vi "TeachAndPlay.vi"() -> ()   [LabVIEW 2013]
uses:
  ROS/Code/JointPositions.ctl
  ROS/Code/SubVIs/BaxterSide.ctl
  ROS/Code/SubVIs/BaxterButtons.ctl
  BaxterVIs/Command_Joint_Angles_cluster.vi
panel:
  in  "Idle Ctr 2":i32=1070
  in  "ITB Cluster":cluster{i16, i16, i16, i16}
  in  "Idle Ctr":i32=411
  in  "Right Path":T2(array[cluster])=[{"Position"={"e0"=0.0, "e1"=90.0, "s0"=50.0, "s1"=0.0, "w0"=0.0, "w1"=0.0, "w2"=0.0}, "Name"="Position0", "Gripper"=FALSE}, {"Position"={"e0"=0.0, "e1"=90.0, "s0"=30.0, "s1"=0.0, "w0"=0.0, "w1"=0.0, "w2"=0.0}, "Name"="Drop", "Gripper"=FALSE}] {"Position"."w2" scale=-175.25..175.25; "Position"."w1" scale=-90.0..120.0; "Position"."w0" scale=-175.25..175.25; "Position"."e1" scale=-3.0..150.0; "Position"."e0" scale=-173.5..173.5; "Position"."s1" scale=-123.0..60.0; "Position"."s0" scale=-141.0..51.0}
  in  "Functions":i32[](listbox)=[0, 1, 4, 5]
  out "Gripper State":bool
  in  "Left Path":T2(array[cluster])=[{"Position"={"e0"=0.0, "e1"=90.0, "s0"=-30.0, "s1"=0.0, "w0"=0.0, "w1"=0.0, "w2"=0.0}, "Name"="Position0", "Gripper"=FALSE}, {"Position"={"e0"=0.0, "e1"=90.0, "s0"=-50.0, "s1"=0.0, "w0"=0.0, "w1"=0.0, "w2"=0.0}, "Name"="Drop", "Gripper"=FALSE}] {"Position"."w2" scale=-175.25..175.25; "Position"."w1" scale=-90.0..120.0; "Position"."w0" scale=-175.25..175.25; "Position"."e1" scale=-3.0..150.0; "Position"."e0" scale=-173.5..173.5; "Position"."s1" scale=-123.0..60.0; "Position"."s0" scale=-141.0..51.0}
  in  "Tab":T3(tab)=enum."Play"
  in  "New Path?":bool
  out "Last Activity":string="Initializing"
  in  "Side":T4=enum."right"
  in  "New Path?":bool
  out "Last Activity":string="Initializing"
  in  "Settle":bool
  in  "Resend Right":bool
  in  "Resend Left":bool
  in  "Tolerance":dbl=1.0
  in  "Settle Time":u32=1000
  in  "Loop?":bool
  in  "Execution":T5(radio)
  in  "Left Step":i32
  in  "Right Step":i32
  in  "Same?":bool
  in  "right save path":path=path "C:/Program Files/Labview/user.lib/ROSforLV_0.1/Devices/Baxter/Baxter Examples/Paths/Tsai2RightW2.csv"
  in  "left save path":path=path "C:/Program Files/Labview/user.lib/ROSforLV_0.1/Devices/Baxter/Baxter Examples/Paths/TsaiLeftW2.csv"
  in  "Save":bool
  in  "left load file":path=path "C:/Program Files/Labview/user.lib/ROSforLV_0.1/Devices/Baxter/Baxter Examples/Paths/TsaiLeftS0.csv"
  in  "Load":bool
  in  "right load file":path=path "C:/Program Files/Labview/user.lib/ROSforLV_0.1/Devices/Baxter/Baxter Examples/Paths/Tsai2RightS0.csv"
  in  "stop":bool
  # "Not yet"
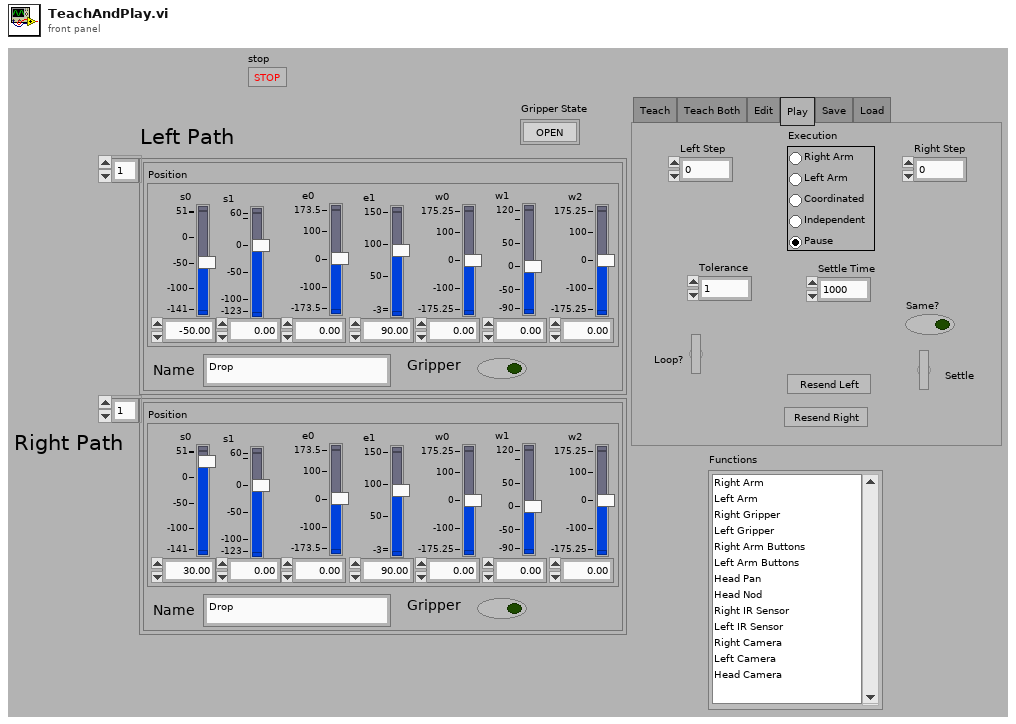
[diagram p1: front panel]
types:
  T1 = typedef "JointPositions.ctl" = cluster{"e0":dbl, "e1":dbl, "s0":dbl, "s1":dbl, "w0":dbl, "w1":dbl, "w2":dbl}
  T2 = cluster{"Position":T1, "Name":string, "Gripper":bool}[]
  T3 = enum32{"Teach", "Teach Both", "Edit", "Play", "Save", "Load"}
  T4 = typedef "BaxterSide.ctl" = enum16{"left", "right"}
  T5 = enum32{"Pause", "Right Arm", "Left Arm", "Coordinated", "Independent"}
  T6 = cluster{"Positions":T1, "Name":string, "Gripper":bool}
  T7 = enum16{"open", "replace", "create", "open or create", "replace or create", "replace or create with confirmation"}
  T8 = typedef "BaxterButtons.ctl" = u16
  T9 = cluster{"Cancel":bool, "OK":bool, "Show":bool, "Wheel":u8}
  T10 = cluster{"Positions":T1, "Name":string, "Gripper":bool}[]
  T11 = cluster{"Position":T1, "Name":string, "Gripper":bool}
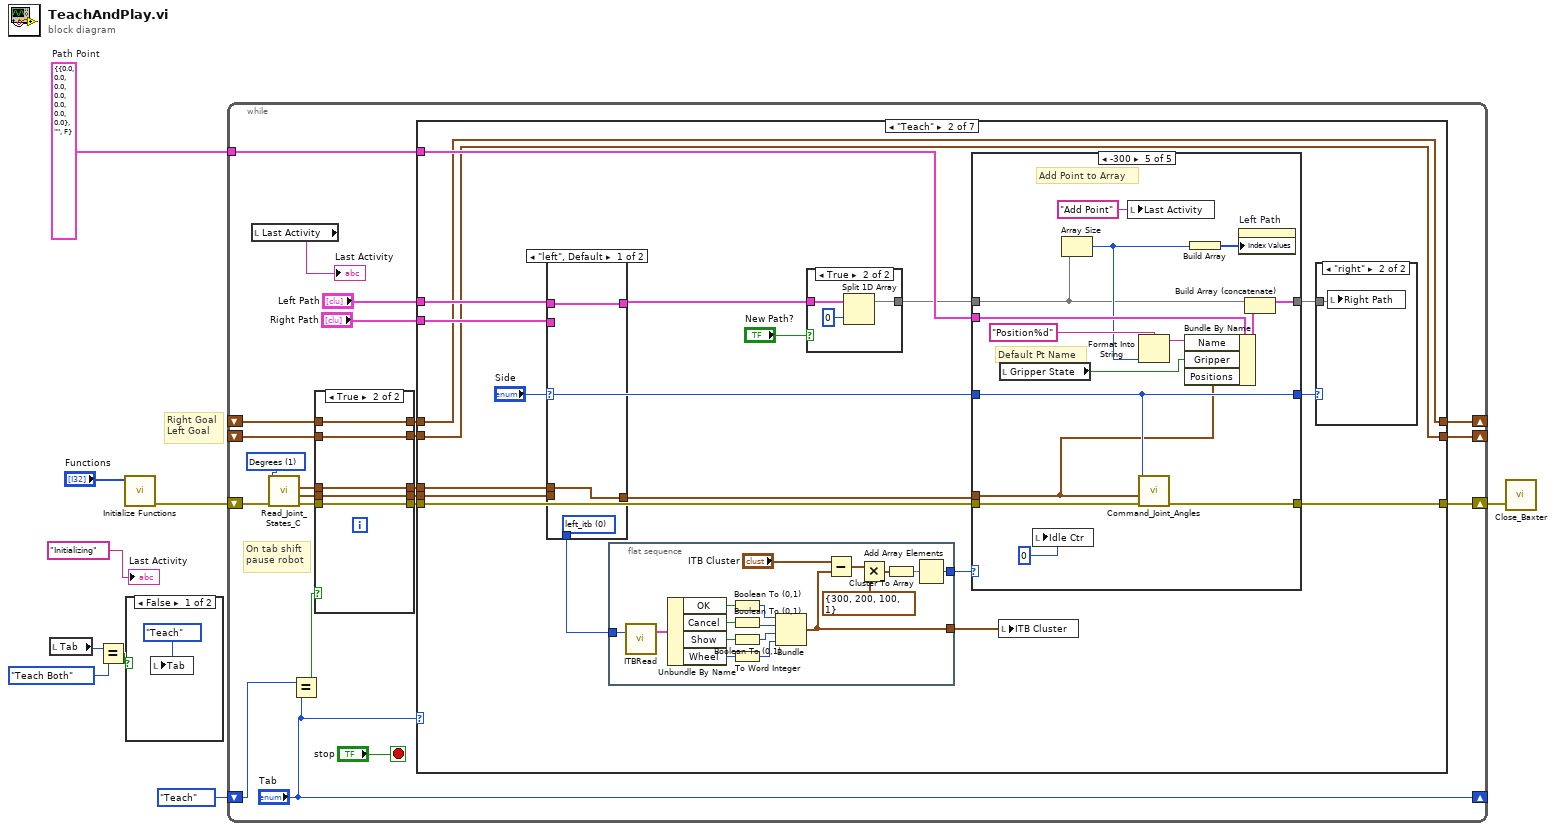
[diagram p0: block diagram]
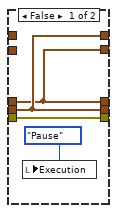
[diagram p3: hidden frame]
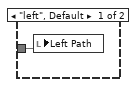
[diagram p5: hidden frame]
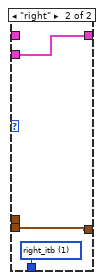
[diagram p6: hidden frame]
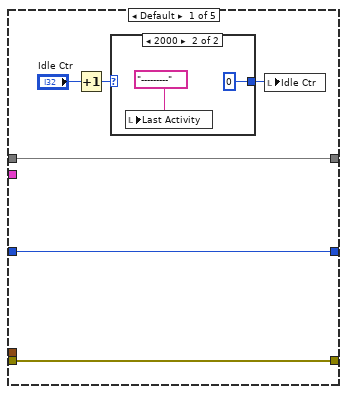
[diagram p8: hidden frame]
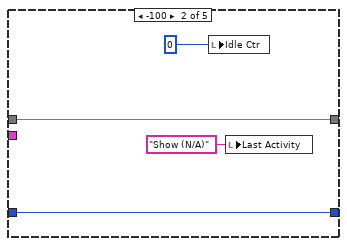
[diagram p10: hidden frame]
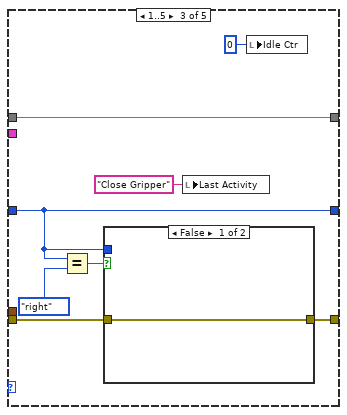
[diagram p11: hidden frame]
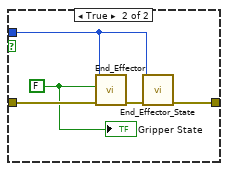
[diagram p12: hidden frame]
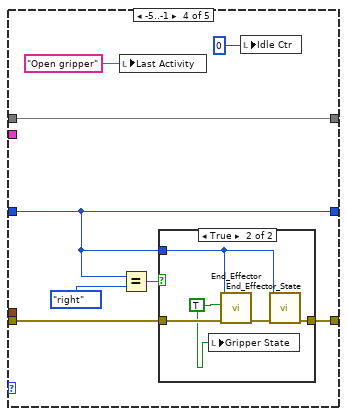
[diagram p13: hidden frame]
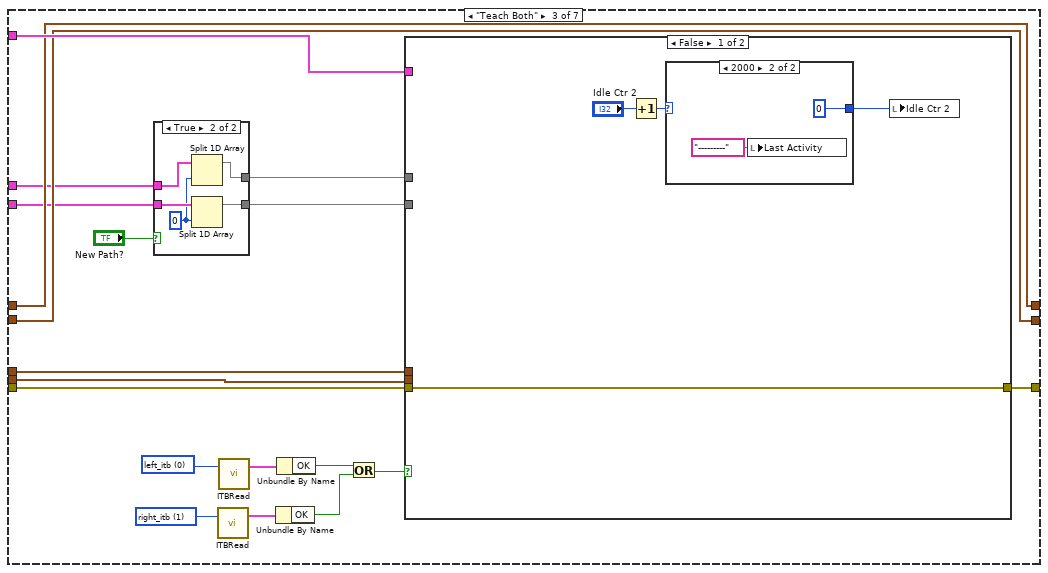
[diagram p15: hidden frame]
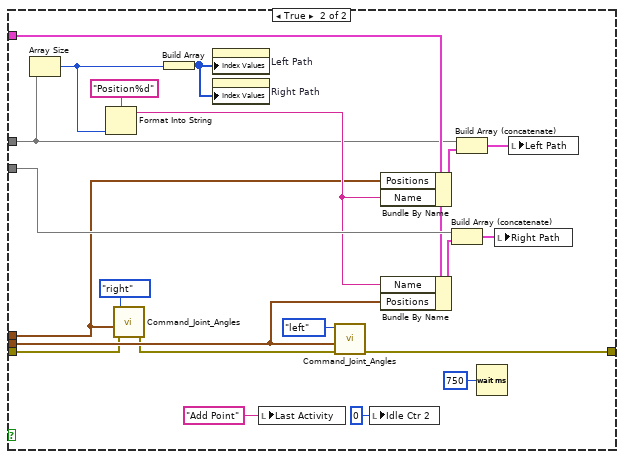
[diagram p18: hidden frame]
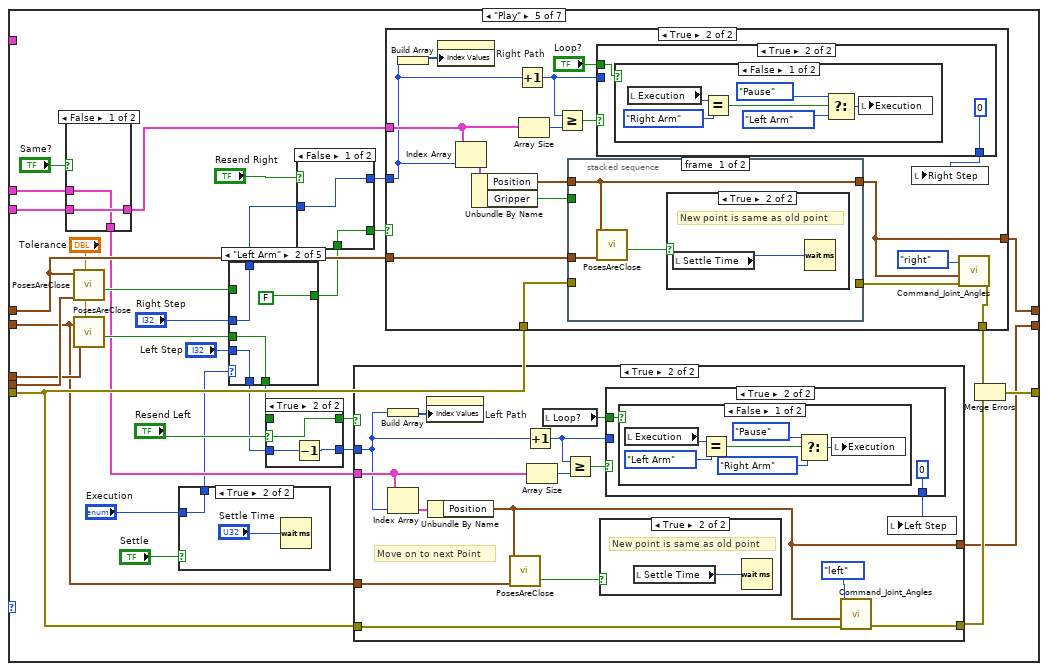
[diagram p20: hidden frame]
diagram:
  w8 = T6 {"Positions"={"e0"=0.0, "e1"=0.0, "s0"=0.0, "s1"=0.0, "w0"=0.0, "w1"=0.0, "w2"=0.0}, "Name"="", "Gripper"=FALSE}  # Path Point
  # "Right Goal\nLeft Goal"
  n1 = local read "Tab"() -> (w4:T3)
  n2 = Equal?(x=w4, y=T3."Teach Both") -> (x = y?=w2:bool)
  n3 = call "Initialize Functions.vi"("Functions"="Functions") -> ("error out"=w9:errorcluster)  [unwired: 10 in]
  n4 = case shown="False" w2 {
    frame False {
      n5 = local write "Tab"(T3."Teach" ("Tab")) -> ()
    }
    frame True {
    }
  }
  n6 = while {
    tunnel: w8 -> [w33]
    shift-right: [w32] -> w7
    shift-left: w9 -> [w30]
    shift-right: ["Tab"] -> _
    shift-left: enum32{"Teach", "Edit", "Run", "Save", "Load"}."Teach" ("Tab") -> [w29]
    shift-right: [w14] -> _
    shift-left: _ -> [w21]
    shift-right: [w12] -> _
    shift-left: _ -> [w15]
    stop <- "stop" stop-if-true
    w31 = u16 1 items=["Radians", "Degrees"] ("Units (Rad)")
    # "On tab shift\npause robot"
    n7 = local read "Last Activity"() -> (→"Last Activity":string)
    n8 = call "Read_Joint_States_C.vi"("error in"=w30, "Units (deg)"=w31) -> ("error out"=w26:errorcluster, "right Positions"=w25:T1, "left Positions"=w17:T1)  [unwired: 3 in, 1 out]
    n9 = Equal?(x=w29, y="Tab") -> (x = y?=w27:bool)
    n10 = case shown="True" w27 {
      tunnel: w26 -> [w36 w42]
      tunnel: w25 -> [w37 w40]
      tunnel: [w36 w42] -> w24
      tunnel: [w37 w40] -> w23
      tunnel: w21 -> [_ w41]
      tunnel: [w37 w41] -> w20
      tunnel: w17 -> [w35 w39]
      tunnel: [w35 w39] -> w16
      tunnel: [w35 w38] -> w13
      tunnel: w15 -> [_ w38]
      frame False {
        n11 = local write "Execution"(T5."Pause" ("Execution")) -> ()
      }
      frame True {
      }
    }
    n12 = case shown="\"Teach\"" "Tab" {
      tunnel: w33 -> [_ w63 w168 _ _ _ w402]
      tunnel: w24 -> [w45 w62 w167 w204 w239 _ _]
      tunnel: [w45 w61 w166 w204 w235 _ _] -> w32
      tunnel: w23 -> [_ w51 w161 _ w236 _ _]
      tunnel: [w44 w49 w164 w206 w237 w350 w399] -> w14
      tunnel: w20 -> [w44 w49 w164 w206 w238 w350 w399]
      tunnel: "Left Path" -> [_ w55 w159 _ w213 w352 _]
      tunnel: "Right Path" -> [_ w56 w160 _ w210 w348 _]
      tunnel: w16 -> [_ w52 w150 _ w220 _ _]
      tunnel: w13 -> [w43 w48 w163 w205 w219 w349 w400]
      tunnel: [w43 w48 w163 w205 w229 w349 w400] -> w12
      frame Default {
      }
      frame "Teach" {
        n13 = case shown="\"left\", Default" "Side" {
          tunnel: [w86 w89] -> w57
          tunnel: w56 -> [_ w89]
          tunnel: w55 -> [w86 _]
          tunnel: [w85 w88] -> w54
          tunnel: [w84 w87] -> w53
          tunnel: w52 -> [w84 _]
          tunnel: w51 -> [_ w87]
          frame "left", Default {
            w85 = T8 0 items=["left_itb", "right_itb", "torso_left_itb", "torso_right_itb"] ("Component")
          }
          frame "right" {
            w88 = T8 1 items=["left_itb", "right_itb", "torso_left_itb", "torso_right_itb"] ("Component")
          }
        }
        n14 = flat-sequence {
          tunnel: [w70] -> w64
          tunnel: w54 -> [w69]
          tunnel: [w68] -> w50
          frame #0 {
            n15 = call "ITBRead.vi"("Component"=w69) -> ("ITB"=w83:T9)  [unwired: 2 in, 1 out]
            n16 = Unbundle By Name(w83) -> ("OK"=w82:bool, "Cancel"=w81:bool, "Show"=w80:bool, "Wheel"=w78:u8)
            n17 = Boolean To (0,1)(Boolean=w82) -> (0, 1=w79:i16)
            n18 = Boolean To (0,1)(Boolean=w81) -> (0, 1=w76:i16)
            n19 = Boolean To (0,1)(Boolean=w80) -> (0, 1=w77:i16)
            n20 = To Word Integer(number=w78) -> (16bit integer=w75:i16)
            n21 = Bundle(w79, w76, w77, w75) -> (w68:cluster{i16, i16, i16, i16})  [unwired: 1 in]
            n22 = Subtract(x="ITB Cluster", y=w68) -> (x-y=w74:cluster{i16, i16, i16, i16})
            n23 = Multiply(x=w74, y=cluster{i16, i16, i16, i16} {300, 200, 100, 1}) -> (x*y=w72:cluster{i16, i16, i16, i16})
            n24 = Cluster To Array(cluster=w72) -> (array=w71:i16[])
            n25 = Add Array Elements(numeric array=w71) -> (sum=w70:i16)
          }
        }
        n26 = case shown="True" "New Path?" {
          tunnel: w57 -> [w90 w92]
          tunnel: [w90 w91] -> w59
          frame False {
          }
          frame True {
            n27 = Split 1D Array(array=w92, index=0) -> (first subarray=w91:T2)  [unwired: 1 out]
          }
        }
        n28 = case shown="-300" w64 {
          tunnel: w63 -> [_ _ _ _ w148]
          tunnel: w62 -> [w99 _ w114 w128 w141]
          tunnel: [w99 _ w112 w127 w147] -> w61
          tunnel: w53 -> [_ _ _ _ w135]
          tunnel: w59 -> [w95 w103 w109 w123 w140]
          tunnel: "Side" -> [w94 w104 w107 w121 w136]
          tunnel: [w95 w103 w109 w123 w137] -> w47
          tunnel: [w94 w104 w107 w121 w136] -> w46
          frame Default {
            n29 = Increment(x="Idle Ctr") -> (x+1=w98:i32)
            n30 = case shown="2000" w98 {
              selector: w98 -> [w100 _]
              tunnel: [w100 0] -> w96
              frame 0, Default {
              }
              frame 2000 {
                n31 = local write "Last Activity"("---------" ("Last Activity")) -> ()
              }
            }
            n32 = local write "Idle Ctr"(w96) -> ()
          }
          frame -100 {
            n33 = local write "Idle Ctr"(0) -> ()
            n34 = local write "Last Activity"("Show (N/A)" ("Last Activity")) -> ()
          }
          frame 1..5 {
            n35 = Equal?(x=w107, y=BaxterSide."right" ("x")) -> (x = y?=w110:bool)
            n36 = case shown="False" w110 {
              tunnel: w114 -> [w115 w120]
              tunnel: [w115 w118] -> w112
              tunnel: w107 -> [_ w116]
              frame False {
              }
              frame True {
                w117 = FALSE ("Calibrate")
                n37 = call "End_Effector.vi"("error in"=w120, "Open"=w117, "Side"=w116) -> ("error out"=w119:errorcluster)  [unwired: 5 in]
                n38 = call "End_Effector_State.vi"("error in"=w119, "Side"=w116) -> ("error out"=w118:errorcluster)  [unwired: 5 in, 1 out]
                "Gripper State" <- w117
              }
            }
            n39 = local write "Last Activity"("Close Gripper" ("Last Activity")) -> ()
            n40 = local write "Idle Ctr"(0) -> ()
          }
          frame -5..-1 {
            n41 = local write "Last Activity"("Open gripper" ("Last Activity")) -> ()
            n42 = Equal?(x=w121, y=BaxterSide."right" ("x")) -> (x = y?=w124:bool)
            n43 = case shown="True" w124 {
              tunnel: w128 -> [w129 w134]
              tunnel: [w129 w131] -> w127
              tunnel: w121 -> [_ w130]
              frame False {
              }
              frame True {
                w133 = TRUE ("Calibrate")
                n44 = local write "Gripper State"(w133) -> ()
                n45 = call "End_Effector.vi"("error in"=w134, "Open"=w133, "Side"=w130) -> ("error out"=w132:errorcluster)  [unwired: 5 in]
                n46 = call "End_Effector_State.vi"("error in"=w132, "Side"=w130) -> ("error out"=w131:errorcluster)  [unwired: 5 in, 1 out]
              }
            }
            n47 = local write "Idle Ctr"(0) -> ()
          }
          frame -300 {
            # "Default Pt Name"
            # "Add Point to Array"
            n48 = local read "Gripper State"() -> (w139:bool)
            n49 = local write "Idle Ctr"(0) -> ()
            n50 = Array Size(array=w140) -> (size(s)=w143:i32)
            n51 = local write "Last Activity"("Add Point" ("Last Activity")) -> ()
            n52 = Format Into String(format string="Position%d" ("Name"), w143) -> (resulting string=w142:string)  [unwired: 2 in, 1 out]
            n53 = call-poly "Command_Joint_Angles.vi"("error in"=w141, "Arm Angles (degrees)"=w135, "Side"=w136) -> ("error out"=w147:errorcluster)  [unwired: 6 in]
            n54 = Bundle By Name(cluster=w148, "Name"=w142, "Gripper"=w139, "Positions"=w135) -> (w149:T6)
            n55 = Build Array(w143) -> (w145:i32[])
            n56 = property on="Left Path" class="Arr (strict)"("Index Values"=w145) -> ()  [unwired: 2 in, 2 out]
            n57 = Build Array (concatenate)(w140, w149) -> (w137:T10)
          }
        }
        n58 = local write "ITB Cluster"(w50) -> ()
        n59 = case shown="\"right\"" w46 {
          tunnel: w47 -> [w65 w66]
          frame "left", Default {
            n60 = local write "Left Path"(w65) -> ()
          }
          frame "right" {
            n61 = local write "Right Path"(w66) -> ()
          }
        }
      }
      frame "Teach Both" {
        w158 = T8 1 items=["left_itb", "right_itb", "torso_left_itb", "torso_right_itb"] ("Component")
        w155 = T8 0 items=["left_itb", "right_itb", "torso_left_itb", "torso_right_itb"] ("Component")
        n62 = case shown="True" "New Path?" {
          tunnel: w160 -> [w170 w175]
          tunnel: [w170 w174] -> w165
          tunnel: w159 -> [w169 w173]
          tunnel: [w169 w171] -> w151
          frame False {
          }
          frame True {
            w172 = 0 ("index")
            n63 = Split 1D Array(array=w173, index=w172) -> (first subarray=w171:T2)  [unwired: 1 out]
            n64 = Split 1D Array(array=w175, index=w172) -> (first subarray=w174:T2)  [unwired: 1 out]
          }
        }
        n65 = call "ITBRead.vi"("Component"=w158) -> ("ITB"=w157:T9)  [unwired: 2 in, 1 out]
        n66 = call "ITBRead.vi"("Component"=w155) -> ("ITB"=w156:T9)  [unwired: 2 in, 1 out]
        n67 = Unbundle By Name(w157) -> ("OK"=w153:bool)
        n68 = Unbundle By Name(w156) -> ("OK"=w154:bool)
        n69 = Or(x=w154, y=w153) -> (x .or. y?=w152:bool)
        n70 = case shown="False" w152 {
          tunnel: w168 -> [_ w192]
          tunnel: w167 -> [w179 w189]
          tunnel: [w179 w202] -> w166
          tunnel: w161 -> [_ w198]
          tunnel: w165 -> [_ w199]
          tunnel: w151 -> [_ w190]
          tunnel: w150 -> [_ w188]
          frame False {
            n71 = Increment(x="Idle Ctr 2") -> (x+1=w178:i32)
            n72 = case shown="2000" w178 {
              selector: w178 -> [w180 _]
              tunnel: [w180 0] -> w176
              frame 0, Default {
              }
              frame 2000 {
                n73 = local write "Last Activity"("---------" ("Last Activity")) -> ()
              }
            }
            n74 = local write "Idle Ctr 2"(w176) -> ()
          }
          frame True {
            n75 = Array Size(array=w190) -> (size(s)=w200:i32)
            n76 = Format Into String(format string="Position%d" ("Name"), w200) -> (resulting string=w191:string)  [unwired: 2 in, 1 out]
            n77 = call-poly "Command_Joint_Angles.vi"("error in"=w189, "Arm Angles (degrees)"=w188, "Side"=BaxterSide."right") -> ("error out"=w187:errorcluster)  [unwired: 6 in]
            n78 = Build Array(w200) -> (w195:i32[])
            n79 = property on="Left Path" class="Arr (strict)"("Index Values"=w195) -> ()  [unwired: 2 in, 2 out]
            n80 = property on="Right Path" class="Arr (strict)"("Index Values"=w195) -> ()  [unwired: 2 in, 2 out]
            n81 = local write "Last Activity"("Add Point" ("Last Activity")) -> ()
            n82 = call-poly "Command_Joint_Angles.vi"("error in"=w187, "Arm Angles (degrees)"=w198, "Side"=BaxterSide."left") -> ("error out"=w202:errorcluster)  [unwired: 6 in]
            n83 = local write "Idle Ctr 2"(0) -> ()
            n84 = Bundle By Name(cluster=w192, "Positions"=w188, "Name"=w191) -> (w193:T6)
            n85 = Bundle By Name(cluster=w192, "Name"=w191, "Positions"=w198) -> (w203:T6)
            n86 = Build Array (concatenate)(w199, w203) -> (w196:T10)
            n87 = Build Array (concatenate)(w190, w193) -> (w194:T10)
            n88 = Wait (ms)(milliseconds to wait=u32 750) -> ()  [unwired: 1 out]
            n89 = local write "Right Path"(w196) -> ()
            n90 = local write "Left Path"(w194) -> ()
          }
        }
      }
      frame "Edit" {
      }
      frame "Play" {
        n91 = case shown="False" "Same?" {
          tunnel: [w243 w245] -> w212
          tunnel: w213 -> [w243 w245]
          tunnel: [w244 w245] -> w211
          tunnel: w210 -> [w244 _]
          frame False {
          }
          frame True {
          }
        }
        n92 = call "PosesAreClose.vi"("Tolerance"="Tolerance", "Position 2"=w236, "Position"=w238) -> ("Close"=w231:bool)  [unwired: 8 in]
        n93 = call "PosesAreClose.vi"("Tolerance"="Tolerance", "Position 2"=w220, "Position"=w219) -> ("Close"=w230:bool)  [unwired: 8 in]
        n94 = case shown="True" "Settle" {
          tunnel: "Execution" -> [w240 w241]
          tunnel: [w240 w241] -> w207
          frame False {
          }
          frame True {
            n95 = Wait (ms)(milliseconds to wait="Settle Time") -> ()  [unwired: 1 out]
          }
        }
        n96 = case shown="\"Left Arm\"" w207 {
          tunnel: w231 -> [w285 _ w293 w298 _]
          tunnel: w230 -> [_ w289 w294 w297 _]
          tunnel: [w285 FALSE w292 w298 w301] -> w222
          tunnel: [FALSE w289 w292 w297 w301] -> w227
          tunnel: "Right Step" -> [w284 w288 _ w296 w300]
          tunnel: "Left Step" -> [w283 w287 w291 w295 w299]
          tunnel: [w283 w287 w291 w295 w299] -> w216
          tunnel: [w284 w288 w291 w296 w300] -> w215
          frame "Right Arm", Default {
          }
          frame "Left Arm" {
          }
          frame "Coordinated" {
            n97 = And(x=w293, y=w294) -> (x .and. y?=w292:bool)
          }
          frame "Independent" {
          }
          frame "Pause" {
            w301 = FALSE ("Close")
          }
        }
        n98 = case shown="True" "Resend Left" {
          selector: "Resend Left" -> [_ w255]
          tunnel: w227 -> [w252 _]
          tunnel: [w252 w255] -> w226
          tunnel: [w251 w254] -> w225
          tunnel: w216 -> [w251 w253]
          frame False {
          }
          frame True {
            n99 = Decrement(x=w253) -> (x-1=w254:i32)
          }
        }
        n100 = case shown="False" "Resend Right" {
          selector: "Resend Right" -> [_ w250]
          tunnel: [w246 w250] -> w221
          tunnel: w215 -> [w247 w249]
          tunnel: [w247 w248] -> w223
          tunnel: w222 -> [w246 _]
          frame False {
          }
          frame True {
            n101 = Decrement(x=w249) -> (x-1=w248:i32)
          }
        }
        n102 = case shown="True" w226 {
          tunnel: [w257 w264] -> w229
          tunnel: w219 -> [w257 w265]
          tunnel: [w256 w271] -> w233
          tunnel: w212 -> [_ w266]
          tunnel: w239 -> [w256 w263]
          tunnel: w225 -> [_ w261]
          frame False {
            # "Not within Tolerance\nLet Robot Run"
          }
          frame True {
            # "Move on to next Point"
            n103 = Build Array(w261) -> (w259:i32[])
            n104 = Index Array(array=w266, index=w261) -> (element=w272:T11)
            n105 = property on="Left Path" class="Arr (strict)"("Index Values"=w259) -> ()  [unwired: 2 in, 2 out]
            n106 = Unbundle By Name(w272) -> ("Position"=w264:T1)
            n107 = call "PosesAreClose.vi"("Position 2"=w265, "Position"=w264) -> ("Close"=w258:bool)  [unwired: 9 in]
            n108 = Increment(x=w261) -> (x+1=w267:i32)
            n109 = Array Size(array=w266) -> (size(s)=w269:i32)
            n110 = local read "Loop?"() -> (w260:bool)
            n111 = Greater Or Equal?(x=w267, y=w269) -> (x >= y?=w268:bool)
            n112 = case shown="True" w258 {
              frame False {
              }
              frame True {
                # "New point is same as old point"
                n113 = local read "Settle Time"() -> (w273:u32)
                n114 = Wait (ms)(milliseconds to wait=w273) -> ()  [unwired: 1 out]
              }
            }
            n115 = case shown="True" w268 {
              tunnel: w267 -> [w274 _]
              tunnel: [w274 0] -> w262
              tunnel: w260 -> [_ w275]
              frame False {
              }
              frame True {
                n116 = case shown="False" w275 {
                  frame False {
                    n117 = local read "Execution"() -> (w281:T5)
                    n118 = Equal?(x=w281, y=T5."Left Arm" ("Execution")) -> (x = y?=w280:bool)
                    n119 = Select(t=T5."Pause" ("Execution"), s=w280, f=T5."Right Arm" ("Execution")) -> (s? t:f=w279:T5)
                    n120 = local write "Execution"(w279) -> ()
                  }
                  frame True {
                  }
                }
              }
            }
            n121 = call-poly "Command_Joint_Angles.vi"("error in"=w263, "Arm Angles (degrees)"=w264, "Side"=BaxterSide."left") -> ("error out"=w271:errorcluster)  [unwired: 6 in]
            n122 = local write "Left Step"(w262) -> ()
          }
        }
        n123 = case shown="True" w221 {
          tunnel: [w303 w308] -> w237
          tunnel: w238 -> [w303 w309]
          tunnel: w239 -> [w302 w319]
          tunnel: [w302 w317] -> w234
          tunnel: w211 -> [_ w311]
          tunnel: w223 -> [_ w305]
          frame False {
            # "Not within Tolerance\nLet Robot Run"
          }
          frame True {
            n124 = Build Array(w305) -> (w304:i32[])
            n125 = property on="Right Path" class="Arr (strict)"("Index Values"=w304) -> ()  [unwired: 2 in, 2 out]
            n126 = Index Array(array=w311, index=w305) -> (element=w320:T11)
            n127 = Unbundle By Name(w320) -> ("Position"=w310:T1, "Gripper"=w318:bool)
            n128 = Increment(x=w305) -> (x+1=w312:i32)
            n129 = Array Size(array=w311) -> (size(s)=w314:i32)
            n130 = Greater Or Equal?(x=w312, y=w314) -> (x >= y?=w313:bool)
            n131 = stacked-sequence {
              tunnel: w319 -> [_ w328]
              tunnel: w318 -> [_ w326]
              tunnel: [_ w325] -> w316
              tunnel: w310 -> [w322 _]
              tunnel: w309 -> [w323 _]
              tunnel: [w322 _] -> w308
              frame #0 {
                n132 = call "PosesAreClose.vi"("Position 2"=w323, "Position"=w322) -> ("Close"=w321:bool)  [unwired: 9 in]
                n133 = case shown="True" w321 {
                  frame False {
                  }
                  frame True {
                    # "New point is same as old point"
                    n134 = local read "Settle Time"() -> (w324:u32)
                    n135 = Wait (ms)(milliseconds to wait=w324) -> ()  [unwired: 1 out]
                  }
                }
              }
              frame #1 {
                n136 = local read "Gripper State"() -> (w329:bool)
                n137 = Not Equal?(x=w326, y=w329) -> (x != y?=w327:bool)
                n138 = case shown="True" w327 {
                  tunnel: w328 -> [w330 w333]
                  tunnel: w326 -> [_ w332]
                  tunnel: [w330 w331] -> w325
                  frame False {
                  }
                  frame True {
                    n139 = stacked-sequence {
                      tunnel: w333 -> [w336 _]
                      tunnel: w332 -> [w334 _]
                      tunnel: [w335 _] -> w331
                      frame #0 {
                        n140 = local write "Gripper State"(w334) -> ()
                        n141 = call "End_Effector.vi"("error in"=w336, "Open"=w334, "Side"=BaxterSide."right") -> ("error out"=w335:errorcluster)  [unwired: 5 in]
                      }
                      frame #1 {
                        # "Give time for gripper to move"
                        n142 = Wait (ms)(milliseconds to wait=u32 250) -> ()  [unwired: 1 out]
                      }
                    }
                  }
                }
              }
            }
            n143 = case shown="True" w313 {
              tunnel: w312 -> [w339 _]
              tunnel: [w339 0] -> w307
              tunnel: "Loop?" -> [_ w340]
              frame False {
              }
              frame True {
                n144 = case shown="False" w340 {
                  frame False {
                    n145 = local read "Execution"() -> (w346:T5)
                    n146 = Equal?(x=w346, y=T5."Right Arm" ("Execution")) -> (x = y?=w345:bool)
                    n147 = Select(t=T5."Pause" ("Execution"), s=w345, f=T5."Left Arm" ("Execution")) -> (s? t:f=w344:T5)
                    n148 = local write "Execution"(w344) -> ()
                  }
                  frame True {
                  }
                }
              }
            }
            n149 = local write "Right Step"(w307) -> ()
            n150 = call-poly "Command_Joint_Angles.vi"("error in"=w316, "Arm Angles (degrees)"=w308, "Side"=BaxterSide."right") -> ("error out"=w317:errorcluster)  [unwired: 6 in]
          }
        }
        n151 = Merge Errors(w234, w233) -> (w235:errorcluster)
      }
      frame "Save" {
        n152 = case shown="True" "Save" {
          tunnel: w352 -> [_ w364]
          tunnel: w348 -> [_ w355]
          frame False {
          }
          frame True {
            n153 = Open/Create/Replace File(file path (use dialog)="left save path", operation (0:open)=T7."replace or create") -> (refnum out=w363:refnum<file>)  [unwired: 4 in, 2 out]
            n154 = for {
              tunnel: w364 -> [w398] mode=indexing
              tunnel: [w384] -> w362
              tunnel: w363 -> [w383]
              tunnel: [w382] -> w361
              n155 = Unbundle By Name(w398) -> ("Name"=w394:string, "Gripper"=w396:bool, "Position.e0"=w393:dbl, "Position.e1"=w392:dbl, "Position.s0"=w391:dbl, "Position.s1"=w390:dbl, "Position.w0"=w389:dbl, "Position.w1"=w388:dbl, "Position.w2"=w387:dbl)
              n156 = Boolean To (0,1)(Boolean=w396) -> (0, 1=w395:i16)
              n157 = Format Into String(format string="%s,%d,%f,%f,%f,%f,%f,%f,%f\\n", w394, w395, w393, w392, w391, w390, w389, w388, w387) -> (resulting string=w386:string, error out=w385:errorcluster)  [unwired: 2 in]
              n158 = Write to Text File(file (use dialog)=w383, text=w386, error in=w385) -> (refnum out=w382:refnum<file>, error out=w384:errorcluster)  [unwired: 1 in, 1 out]
            }
            n159 = Close File(refnum=w361, error in=w362) -> ()  [unwired: 2 out]
            n160 = Open/Create/Replace File(file path (use dialog)="right save path", operation (0:open)=T7."replace or create") -> (refnum out=w353:refnum<file>)  [unwired: 4 in, 2 out]
            n161 = for {
              tunnel: w355 -> [w381] mode=indexing
              tunnel: [w367] -> w358
              tunnel: w353 -> [w366]
              tunnel: [w365] -> w357
              n162 = Unbundle By Name(w381) -> ("Name"=w377:string, "Gripper"=w379:bool, "Position.e0"=w376:dbl, "Position.e1"=w375:dbl, "Position.s0"=w374:dbl, "Position.s1"=w373:dbl, "Position.w0"=w372:dbl, "Position.w1"=w371:dbl, "Position.w2"=w370:dbl)
              n163 = Boolean To (0,1)(Boolean=w379) -> (0, 1=w378:i16)
              n164 = Format Into String(format string="%s,%d,%f,%f,%f,%f,%f,%f,%f\\n", w377, w378, w376, w375, w374, w373, w372, w371, w370) -> (resulting string=w369:string, error out=w368:errorcluster)  [unwired: 2 in]
              n165 = Write to Text File(file (use dialog)=w366, text=w369, error in=w368) -> (refnum out=w365:refnum<file>, error out=w367:errorcluster)  [unwired: 1 in, 1 out]
            }
            n166 = Close File(refnum=w357, error in=w358) -> ()  [unwired: 2 out]
          }
        }
      }
      frame "Load" {
        n167 = case shown="True" "Load" {
          tunnel: w402 -> [_ w404]
          frame False {
          }
          frame True {
            n168 = Open/Create/Replace File(file path (use dialog)="right load file", operation (0:open)=T7."open") -> (refnum out=w411:refnum<file>, error out=w409:errorcluster)  [unwired: 4 in, 1 out]
            n169 = Open/Create/Replace File(file path (use dialog)="left load file", operation (0:open)=T7."open") -> (refnum out=w421:refnum<file>, error out=w419:errorcluster)  [unwired: 4 in, 1 out]
            n170 = Read from Text File(file (use dialog)=w411, count=-1, error in=w409) -> (refnum out=w410:refnum<file>, text=w406:string[], error out=w408:errorcluster)  [unwired: 1 in, 1 out]
            n171 = Read from Text File(file (use dialog)=w421, count=-1, error in=w419) -> (refnum out=w420:refnum<file>, text=w415:string[], error out=w418:errorcluster)  [unwired: 1 in, 1 out]
            n172 = Close File(refnum=w410, error in=w408) -> (error out=w405:errorcluster)  [unwired: 1 out]
            n173 = Close File(refnum=w420, error in=w418) -> (error out=w414:errorcluster)  [unwired: 1 out]
            n174 = for {
              tunnel: w406 -> [w436] mode=indexing
              tunnel: w404 -> [w439]
              tunnel: [w438] -> w403 mode=indexing
              tunnel: [w437] -> _
              tunnel: w405 -> [w424]
              n175 = Match Pattern(string=w436, regular expression=",") -> (before substring=w433:string, after substring=w434:string)  [unwired: 1 in, 2 out]
              n176 = Scan From String(format string="%d,%f,%f,%f,%f,%f,%f,%f", input string=w434, error in=w424) -> (error out=w437:errorcluster, output 1=w432:i32, output 2=w431:dbl, output 3=w430:dbl, output 4=w429:dbl, output 5=w428:dbl, output 6=w427:dbl, output 7=w426:dbl, output 8=w425:dbl)  [unwired: 9 in, 2 out]
              n177 = Greater Than 0?(x=w432) -> (x > 0?=w440:bool)
              n178 = Bundle By Name(cluster=w439, "Name"=w433, "Gripper"=w440, "Positions.e0"=w431, "Positions.e1"=w430, "Positions.s0"=w429, "Positions.s1"=w428, "Positions.w0"=w427, "Positions.w1"=w426, "Positions.w2"=w425) -> (w438:T6)
            }
            n179 = for {
              tunnel: w415 -> [w454] mode=indexing
              tunnel: w404 -> [w457]
              tunnel: [w456] -> w416 mode=indexing
              tunnel: [w455] -> _
              tunnel: w414 -> [w442]
              n180 = Match Pattern(string=w454, regular expression=",") -> (before substring=w451:string, after substring=w452:string)  [unwired: 1 in, 2 out]
              n181 = Scan From String(format string="%d,%f,%f,%f,%f,%f,%f,%f", input string=w452, error in=w442) -> (error out=w455:errorcluster, output 1=w450:i32, output 2=w449:dbl, output 3=w448:dbl, output 4=w447:dbl, output 5=w446:dbl, output 6=w445:dbl, output 7=w444:dbl, output 8=w443:dbl)  [unwired: 9 in, 2 out]
              n182 = Greater Than 0?(x=w450) -> (x > 0?=w458:bool)
              n183 = Bundle By Name(cluster=w457, "Name"=w451, "Gripper"=w458, "Positions.e0"=w449, "Positions.e1"=w448, "Positions.s0"=w447, "Positions.s1"=w446, "Positions.w0"=w445, "Positions.w1"=w444, "Positions.w2"=w443) -> (w456:T6)
            }
            n184 = local write "Right Path"(w403) -> ()
            n185 = local write "Left Path"(w416) -> ()
          }
        }
      }
    }
  }
  n186 = call "Close_Baxter.vi"("error in"=w7) -> ()  [unwired: 3 in, 1 out]
  "Last Activity" <- "Initializing" ("Last Activity")
